vi "Write Card #.vi"(8 "error in (no error)":errorcluster, 10 "Card #":dbl, 11 "MultiCard Ancestor in":refnum<class "MultiCard Ancestor.lvclass">) -> (0 "error out":errorcluster, 3 "MultiCard Ancestor out":refnum<class "MultiCard Ancestor.lvclass">)   [LabVIEW 2012, in "MultiCard.lvlib" / "MultiCard Ancestor.lvclass"]
uses:
  MultiCard Ancestor.lvclass
  MultiCard Ancestor.lvclass/MultiCard Ancestor.ctl
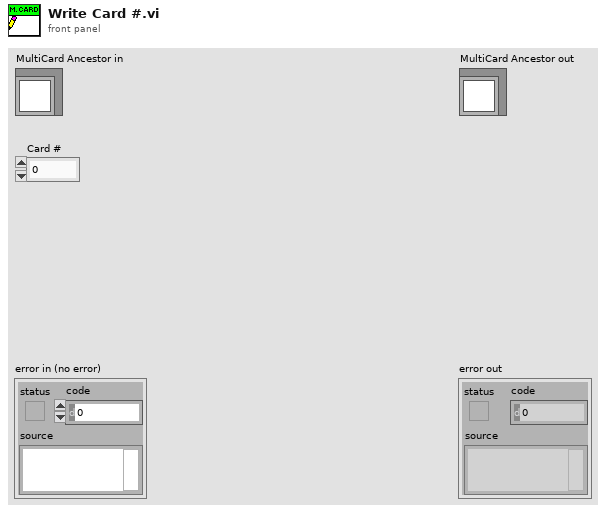
[diagram p1: front panel]
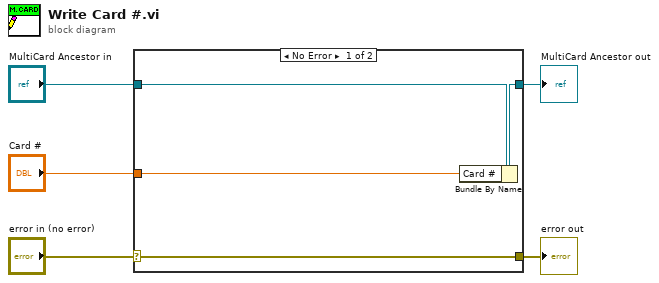
[diagram p0: block diagram]
diagram:
  n1 = case shown="No Error" "error in (no error)" {
    selector: "error in (no error)" -> [w9 w10]
    tunnel: [w9 w10] -> w4
    tunnel: [w7 w11] -> w2
    tunnel: "MultiCard Ancestor in" -> [w8 w11]
    tunnel: "Card #" -> [w6 _]
    frame No Error {
      n2 = Bundle By Name(cluster=w8, "Card #"=w6) -> (w7:refnum<class "MultiCard Ancestor.lvclass">)
    }
    frame Error {
    }
  }
  "error out" <- w4
  "MultiCard Ancestor out" <- w2
